vi "test Scheduled Loopback with Disable.vi"(8 "error in":errorcluster, 11 "TestCase in":refnum<class "Octal Loopback.lvclass">) -> (0 "error out":errorcluster, 3 "TestCase out":refnum<class "Octal Loopback.lvclass">)   [LabVIEW 2020, in "Octal Loopback.lvclass"]
uses:
  Octal Loopback.lvclass
  C:/Program Files (x86)/National Instruments/LabVIEW 2020/vi.lib/NI/VeriStand Custom Device Testing Tools/VeriStandTestCase/VeriStandTestCase.lvclass
  <vilib>/numeric/Random Number (Range) U64.vi
  <vilib>/numeric/sub_Random U32.vi
  <vilib>/NI VeriStand/Execution/Workspace/NI VeriStand - Set Multiple Channel Values.vi
  <vilib>/addons/_JKI Toolkits/VI Tester/TestCase.llb/TestCase.lvclass
  <vilib>/NI/VeriStand Custom Device Testing Tools/VeriStandTestUtilities/VeriStandTestUtilities.lvlib
  <vilib>/NI VeriStand/Execution/Workspace/NI_VS Workspace ExecutionAPI.lvlib
  C:/Program Files (x86)/National Instruments/LabVIEW 2020/vi.lib/addons/_JKI Toolkits/VI Tester/TestCase.llb/TestCase.lvclass
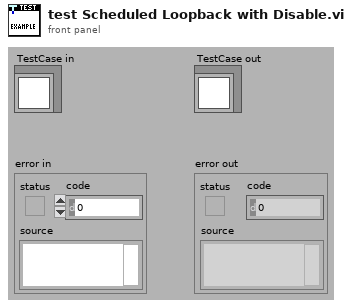
[diagram p1: front panel]
types:
  T1 = typedef "NI_VS Workspace ExecutionAPI.lvlib/WorkspaceAPI.ctl" = refnum<k24>
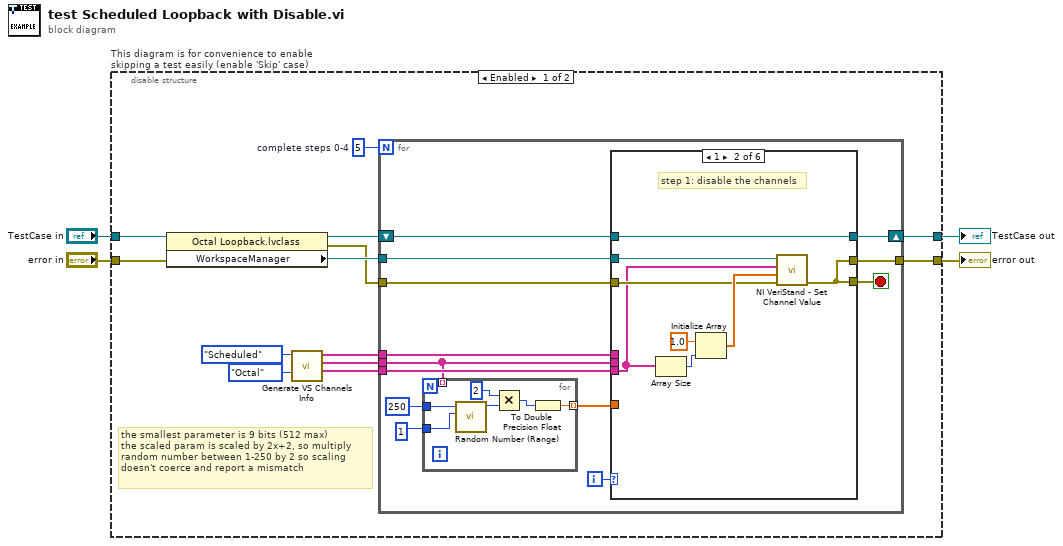
[diagram p0: block diagram]
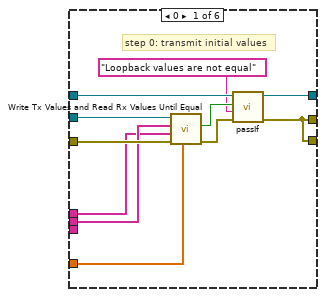
[diagram p2: hidden frame]
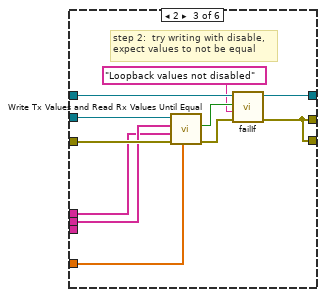
[diagram p3: hidden frame]
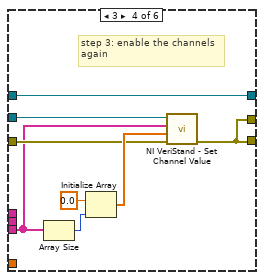
[diagram p4: hidden frame]
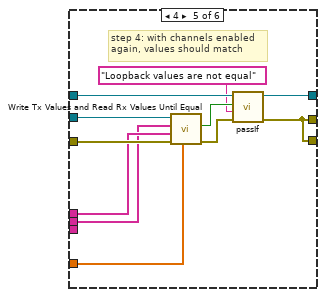
[diagram p5: hidden frame]
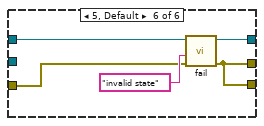
[diagram p6: hidden frame]
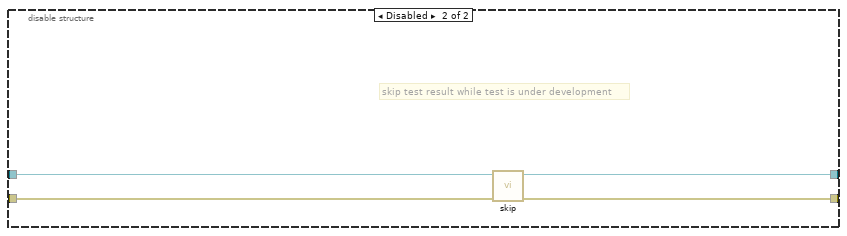
[diagram p7: hidden frame]
diagram:
  n1 = disable-structure "This diagram is for convenience to enable skipping a test easily (enable 'Skip' case)" shown="Enabled" {
    disable-tunnel: "TestCase in" -> [w13 w94]
    disable-tunnel: [w11 w92] -> w1
    disable-tunnel: [w10 w93] -> w3
    disable-tunnel: "error in" -> [w12 w91]
    frame Enabled {
      w7 = 5  # complete steps 0-4
      # "the smallest parameter is 9 bits (512 max)\nthe scaled param is scaled by 2x+2, so multiply \nrandom number between 1-250 by 2 so scaling\ndoesn't coerce and report a mismatch"
      n2 = property class="Octal Loopback.lvclass"(reference=w13, error in=w12) -> (reference out=w14:refnum<class "Octal Loopback.lvclass">, error out=w15:errorcluster, "WorkspaceManager"=w16:T1)
      n3 = call "Generate VS Channels Info.vi"("Label Format (Decimal)"=enum16{"Decimal", "Octal"}."Octal", "Transfer Type"=enum16{"Acyclic", "Scheduled"}."Scheduled") -> ("Tx Disable Channels Array"=w8:string[], "Tx Channels Array"=w9:string[], "Rx Channels Array"=w17:string[])  [unwired: 5 in, 2 out]
      n4 = for {
        N: w7 -> [_]
        tunnel: w17 -> [w30]
        tunnel: w16 -> [w29]
        tunnel: w15 -> [w28]
        tunnel: w9 -> [w18]
        shift-right: [w26] -> w11
        shift-left: w14 -> [w27]
        tunnel: [w25] -> w10
        tunnel: w8 -> [w22]
        i -> [w24]
        stop <- w23 stop-if-true
        n5 = for {
          tunnel: [w35] -> w21 mode=indexing
          tunnel: u64 250 ("upper bound (100)") -> [w34]
          tunnel: u64 1 ("upper bound (100)") -> [w33]
          tunnel: w18 -> [_] mode=indexing
          n6 = call-poly <vilib>:"Random Number (Range).vi"("lower bound (0)"=w33, "upper bound (100)"=w34) -> ("number"=w36:u64)  [unwired: 9 in]
          n7 = Multiply(x=u64 2, y=w36) -> (x*y=w32:u64)
          n8 = To Double Precision Float(number=w32) -> (double precision float=w35:dbl)
        }
        n9 = case shown="1" w24 {
          tunnel: w30 -> [w38 _ w57 _ w77 _]
          tunnel: w29 -> [w47 w51 w66 w70 w85 _]
          tunnel: w28 -> [w46 w50 w65 w69 w84 w87]
          tunnel: w27 -> [w44 w55 w63 w74 w82 w89]
          tunnel: [w43 w55 w62 w74 w81 w90] -> w26
          tunnel: [w40 w49 w59 w68 w78 w86] -> w25
          tunnel: w18 -> [w39 _ w58 _ w76 _]
          tunnel: [w40 w49 w59 w68 w78 w86] -> w23
          tunnel: w22 -> [_ w48 _ w67 _ _]
          tunnel: w21 -> [w37 _ w56 _ w75 _]
          frame 0 {
            # "step 0: transmit initial values"
            n10 = call <vilib>:"Write Tx Values and Read Rx Values Until Equal.vi"("Tx values"=w37, "error in"=w46, "Rx aliases"=w38, "Tx aliases"=w39, "workspace manager in"=w47) -> ("error out"=w45:errorcluster, "values equal"=w42:bool)  [unwired: 4 in, 1 out]
            n11 = call-dynamic "passIf.vi"("error in (no error)"=w45, "message (\"\")"="Loopback values are not equal" ("message (\"\")"), "pass"=w42, "TestCase in"=w44) -> ("error out"=w40:errorcluster, "TestCase out"=w43:refnum<class "Octal Loopback.lvclass">)  [unwired: 6 in]
          }
          frame 1 {
            # "step 1: disable the channels"
            n12 = Array Size(array=w48) -> (size(s)=w54:i32)
            n13 = Initialize Array(1.0 ("element"), w54) -> (w52:dbl[])
            n14 = call-poly <vilib>:"NI VeriStand - Set Channel Value.vi"("error in (no error)"=w50, "Values"=w52, "Channels"=w48, "WorkspaceManager in"=w51) -> ("error out"=w49:errorcluster)  [unwired: 6 in, 1 out]
          }
          frame 2 {
            # "step 2:  try writing with disable,\nexpect values to not be equal"
            n15 = call <vilib>:"Write Tx Values and Read Rx Values Until Equal.vi"("Tx values"=w56, "error in"=w65, "Rx aliases"=w57, "Tx aliases"=w58, "workspace manager in"=w66) -> ("error out"=w64:errorcluster, "values equal"=w61:bool)  [unwired: 4 in, 1 out]
            n16 = call-dynamic "failIf.vi"("error in (no error)"=w64, "message (\"\")"="Loopback values not disabled" ("message (\"\")"), "fail"=w61, "TestCase in"=w63) -> ("error out"=w59:errorcluster, "TestCase out"=w62:refnum<class "Octal Loopback.lvclass">)  [unwired: 6 in]
          }
          frame 3 {
            # "step 3: enable the channels\nagain"
            n17 = Array Size(array=w67) -> (size(s)=w73:i32)
            n18 = Initialize Array(0.0 ("element"), w73) -> (w71:dbl[])
            n19 = call-poly <vilib>:"NI VeriStand - Set Channel Value.vi"("error in (no error)"=w69, "Values"=w71, "Channels"=w67, "WorkspaceManager in"=w70) -> ("error out"=w68:errorcluster)  [unwired: 6 in, 1 out]
          }
          frame 4 {
            # "step 4: with channels enabled\nagain, values should match"
            n20 = call <vilib>:"Write Tx Values and Read Rx Values Until Equal.vi"("Tx values"=w75, "error in"=w84, "Rx aliases"=w77, "Tx aliases"=w76, "workspace manager in"=w85) -> ("error out"=w83:errorcluster, "values equal"=w80:bool)  [unwired: 4 in, 1 out]
            n21 = call-dynamic "passIf.vi"("error in (no error)"=w83, "message (\"\")"="Loopback values are not equal" ("message (\"\")"), "pass"=w80, "TestCase in"=w82) -> ("error out"=w78:errorcluster, "TestCase out"=w81:refnum<class "Octal Loopback.lvclass">)  [unwired: 6 in]
          }
          frame 5, Default {
            n22 = call-dynamic "fail.vi"("error in (no error)"=w87, "message (\"\")"="invalid state" ("message (\"\")"), "TestCase in"=w89) -> ("error out"=w86:errorcluster, "TestCase out"=w90:refnum<class "Octal Loopback.lvclass">)  [unwired: 7 in]
          }
        }
      }
    }
    frame Disabled {
      # "skip test result while test is under development"
      n23 = call <vilib>:"skip.vi"("error in (no error)"=w91, "TestCase in"=w94) -> ("error out"=w93:errorcluster, "TestCase out"=w92:refnum<class "Octal Loopback.lvclass">)  [unwired: 8 in]
    }
  }
  "error out" <- w3
  "TestCase out" <- w1
